vi "RichToFlatnixnet_grpc_GetPropertyResponse.vi"(5 "OutputClusterType":T1, 11 "InputCluster":T9) -> (3 "OutputCluster":T1)   [LabVIEW 2025, in "xnet-grpc_client.lvlib"]
uses:
  nixnet_grpc_GetPropertyResponse.ctl
  nixnet_grpc_GetPropertyResponse_property_value/nixnet_grpc_GetPropertyResponse_property_value.lvclass
  nixnet_grpc_GetPropertyResponse_Flat.ctl
  nixnet_grpc_U32Array_Flat.ctl
  nidevice_grpc_Session_Flat.ctl
  nixnet_grpc_DbRefArray_Flat.ctl
  nixnet_grpc_DeviceRefArray_Flat.ctl
  nixnet_grpc_InterfaceRefArray_Flat.ctl
  nixnet_grpc_EptRxFilterArray_Flat.ctl
  nixnet_grpc_EptRxFilter_Flat.ctl
  xnet-grpc_client.lvlib
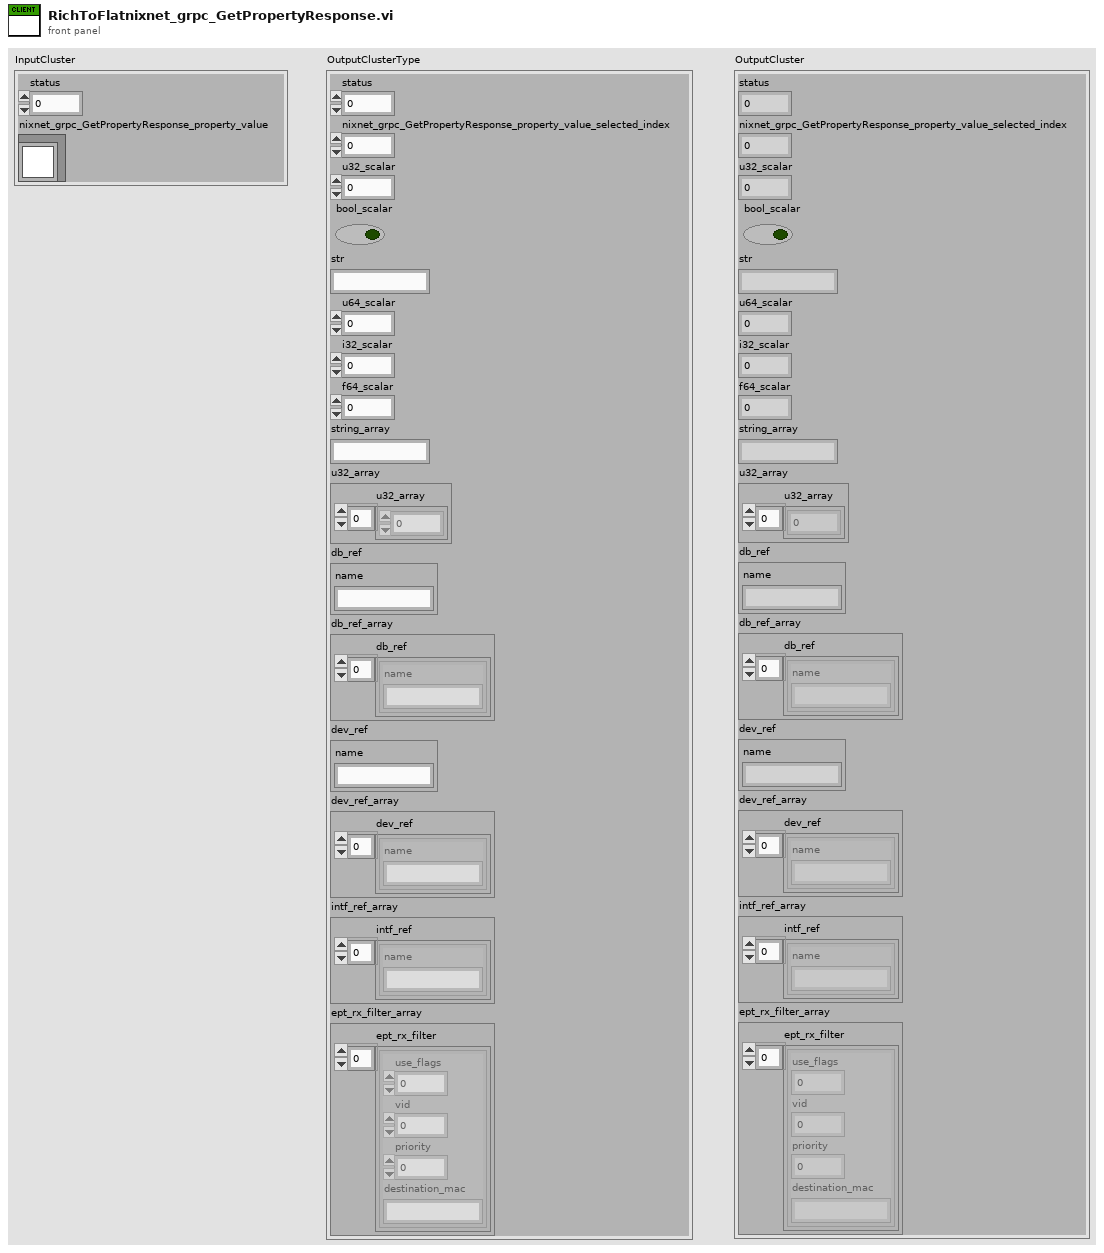
[diagram p1: front panel]
types:
  T1 = typedef "xnet-grpc_client.lvlib/nixnet_grpc_GetPropertyResponse_Flat.ctl" = cluster{"status":i32, "nixnet_grpc_GetPropertyResponse_property_value_selected_index":i32, "u32_scalar":u32, "bool_scalar":bool, "str":string, "u64_scalar":u64, "i32_scalar":i32, "f64_scalar":dbl, "string_array":string, "u32_array":T2, "db_ref":T3, "db_ref_array":T4, "dev_ref":T3, "dev_ref_array":T5, "intf_ref_array":T6, "ept_rx_filter_array":T7}
  T2 = typedef "xnet-grpc_client.lvlib/nixnet_grpc_U32Array_Flat.ctl" = cluster{"u32_array":u32[]}
  T3 = typedef "xnet-grpc_client.lvlib/nidevice_grpc_Session_Flat.ctl" = cluster{"name":string}
  T4 = typedef "xnet-grpc_client.lvlib/nixnet_grpc_DbRefArray_Flat.ctl" = cluster{"db_ref":T3[]}
  T5 = typedef "xnet-grpc_client.lvlib/nixnet_grpc_DeviceRefArray_Flat.ctl" = cluster{"dev_ref":T3[]}
  T6 = typedef "xnet-grpc_client.lvlib/nixnet_grpc_InterfaceRefArray_Flat.ctl" = cluster{"intf_ref":T3[]}
  T7 = typedef "xnet-grpc_client.lvlib/nixnet_grpc_EptRxFilterArray_Flat.ctl" = cluster{"ept_rx_filter":T8[]}
  T8 = typedef "xnet-grpc_client.lvlib/nixnet_grpc_EptRxFilter_Flat.ctl" = cluster{"use_flags":u32, "vid":u32, "priority":u32, "destination_mac":string}
  T9 = typedef "xnet-grpc_client.lvlib/nixnet_grpc_GetPropertyResponse.ctl" = cluster{"status":i32, "nixnet_grpc_GetPropertyResponse_property_value":refnum<class "nixnet_grpc_GetPropertyResponse_property_value.lvclass">}
  T10 = typedef "xnet-grpc_client.lvlib/nixnet_grpc_U32Array.ctl" = cluster{"u32_array":u32[]}
  T11 = typedef "xnet-grpc_client.lvlib/nidevice_grpc_Session.ctl" = cluster{"name":string}
  T12 = typedef "xnet-grpc_client.lvlib/nixnet_grpc_DbRefArray.ctl" = cluster{"db_ref":T11[]}
  T13 = typedef "xnet-grpc_client.lvlib/nixnet_grpc_DeviceRefArray.ctl" = cluster{"dev_ref":T11[]}
  T14 = typedef "xnet-grpc_client.lvlib/nixnet_grpc_InterfaceRefArray.ctl" = cluster{"intf_ref":T11[]}
  T15 = typedef "xnet-grpc_client.lvlib/nixnet_grpc_EptRxFilterArray.ctl" = cluster{"ept_rx_filter":T16[]}
  T16 = typedef "xnet-grpc_client.lvlib/nixnet_grpc_EptRxFilter.ctl" = cluster{"use_flags":u32, "vid":u32, "priority":u32, "destination_mac":string}
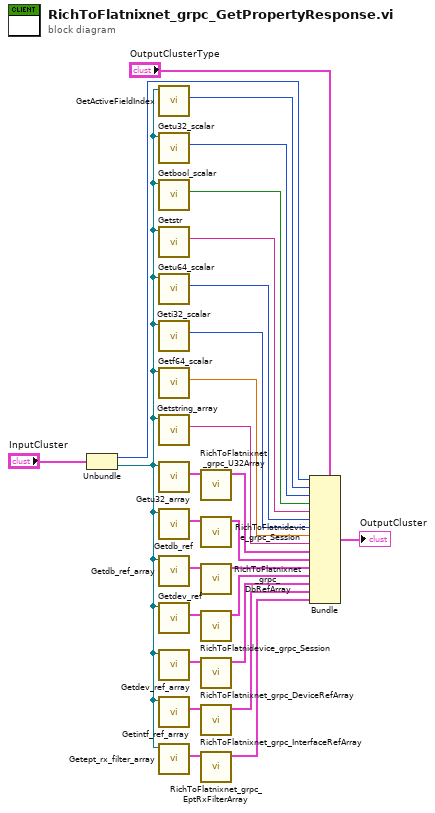
[diagram p0: block diagram]
diagram:
  n1 = Unbundle "Unbundle"("InputCluster") -> ("status"=w24:i32, "nixnet_grpc_GetPropertyResponse_property_value"=w23:refnum<class "nixnet_grpc_GetPropertyResponse_property_value.lvclass">)
  n2 = call "GetActiveFieldIndex.vi"("OneOfTemplate in"=w23) -> ("Active Field Index"=w22:i32)  [unwired: 8 in, 2 out]
  n3 = call "Getu32_scalar.vi"("OneOfTemplate in"=w23) -> ("Get_Val"=w21:u32)  [unwired: 8 in, 2 out]
  n4 = call "Getbool_scalar.vi"("OneOfTemplate in"=w23) -> ("Get_Val"=w20:bool)  [unwired: 8 in, 2 out]
  n5 = call "Getstr.vi"("OneOfTemplate in"=w23) -> ("Get_Val"=w19:string)  [unwired: 8 in, 2 out]
  n6 = call "Getu64_scalar.vi"("OneOfTemplate in"=w23) -> ("Get_Val"=w18:u64)  [unwired: 8 in, 2 out]
  n7 = call "Geti32_scalar.vi"("OneOfTemplate in"=w23) -> ("Get_Val"=w17:i32)  [unwired: 8 in, 2 out]
  n8 = call "Getf64_scalar.vi"("OneOfTemplate in"=w23) -> ("Get_Val"=w16:dbl)  [unwired: 8 in, 2 out]
  n9 = call "Getstring_array.vi"("OneOfTemplate in"=w23) -> ("Get_Val"=w15:string)  [unwired: 8 in, 2 out]
  n10 = call "Getu32_array.vi"("OneOfTemplate in"=w23) -> ("Get_Val"=w14:T10)  [unwired: 8 in, 2 out]
  n11 = call "Getdb_ref.vi"("OneOfTemplate in"=w23) -> ("Get_Val"=w12:T11)  [unwired: 8 in, 2 out]
  n12 = call "Getdb_ref_array.vi"("OneOfTemplate in"=w23) -> ("Get_Val"=w10:T12)  [unwired: 8 in, 2 out]
  n13 = call "Getdev_ref.vi"("OneOfTemplate in"=w23) -> ("Get_Val"=w8:T11)  [unwired: 8 in, 2 out]
  n14 = call "Getdev_ref_array.vi"("OneOfTemplate in"=w23) -> ("Get_Val"=w6:T13)  [unwired: 8 in, 2 out]
  n15 = call "Getintf_ref_array.vi"("OneOfTemplate in"=w23) -> ("Get_Val"=w4:T14)  [unwired: 8 in, 2 out]
  n16 = call "Getept_rx_filter_array.vi"("OneOfTemplate in"=w23) -> ("Get_Val"=w2:T15)  [unwired: 8 in, 2 out]
  n17 = call "RichToFlatnixnet_grpc_U32Array.vi"("InputCluster"=w14) -> ("OutputCluster"=w13:T2)  [unwired: 10 in]
  n18 = call "RichToFlatnidevice_grpc_Session.vi"("InputCluster"=w12) -> ("OutputCluster"=w11:T3)  [unwired: 10 in]
  n19 = call "RichToFlatnixnet_grpc_DbRefArray.vi"("InputCluster"=w10) -> ("OutputCluster"=w9:T4)  [unwired: 10 in]
  n20 = call "RichToFlatnidevice_grpc_Session.vi"("InputCluster"=w8) -> ("OutputCluster"=w7:T3)  [unwired: 10 in]
  n21 = call "RichToFlatnixnet_grpc_DeviceRefArray.vi"("InputCluster"=w6) -> ("OutputCluster"=w5:T5)  [unwired: 10 in]
  n22 = call "RichToFlatnixnet_grpc_InterfaceRefArray.vi"("InputCluster"=w4) -> ("OutputCluster"=w3:T6)  [unwired: 10 in]
  n23 = call "RichToFlatnixnet_grpc_EptRxFilterArray.vi"("InputCluster"=w2) -> ("OutputCluster"=w1:T7)  [unwired: 10 in]
  n24 = Bundle "Bundle"(cluster="OutputClusterType", "status"=w24, "nixnet_grpc_GetPropertyResponse_property_value_selected_index"=w22, "u32_scalar"=w21, "bool_scalar"=w20, "str"=w19, "u64_scalar"=w18, "i32_scalar"=w17, "f64_scalar"=w16, "string_array"=w15, "u32_array"=w13, "db_ref"=w11, "db_ref_array"=w9, "dev_ref"=w7, "dev_ref_array"=w5, "intf_ref_array"=w3, "ept_rx_filter_array"=w1) -> (→"OutputCluster":T1)
